vi "Pos_Calculate Random Location.vi"(8 "Error":errorcluster, 9 "Window Size":i16, 10 "Border":i16, 11 "Max Size":i16) -> (0 "Error Out":errorcluster, 2 "Bottom Right Out":i16, 3 "Top Left Out":i16)   [LabVIEW 2015]
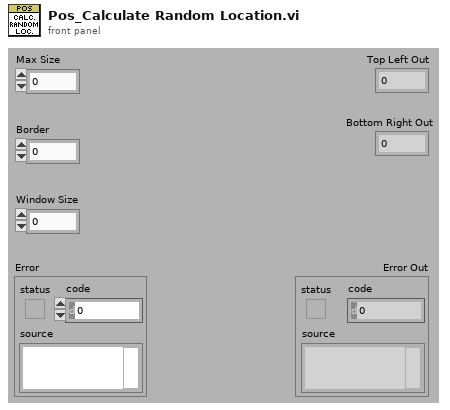
[diagram p1: front panel]
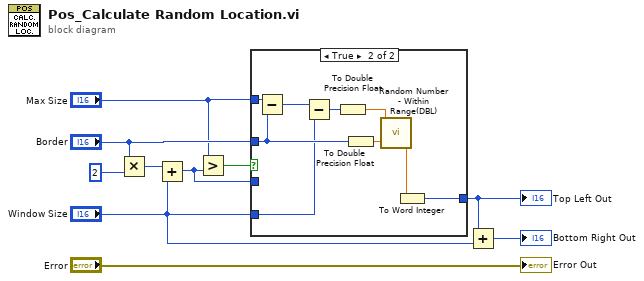
[diagram p0: block diagram]
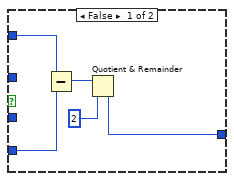
[diagram p2: hidden frame]
diagram:
  n1 = Multiply(x="Border", y=i16 2) -> (x*y=w8:i16)
  n2 = Add(x=w8, y="Window Size") -> (x+y=w4:i16)
  n3 = Greater?(x="Max Size", y=w4) -> (0:w7:bool)
  n4 = case shown="True" w7 {
    tunnel: "Border" -> [_ w22]
    tunnel: "Max Size" -> [w15 w23]
    tunnel: "Window Size" -> [w14 w20]
    tunnel: [w11 w16] -> w2
    tunnel: w4 -> [_ _]
    frame False {
      n5 = Subtract(x=w15, y=w14) -> (x-y=w13:i16)
      n6 = Quotient & Remainder(x=w13, y=i16 2) -> (floor(x/y)=w11:i16)  [unwired: 1 out]
    }
    frame True {
      n7 = Subtract(x=w23, y=w22) -> (x-y=w21:i16)
      n8 = Subtract(x=w21, y=w20) -> (x-y=w19:i16)
      n9 = To Double Precision Float(number=w19) -> (double precision float=w18:dbl)
      n10 = To Double Precision Float(number=w22) -> (double precision float=w24:dbl)
      n11 = call "Random Number - Within Range(DBL).vi"("High (1.00)"=w18, "Low (0.00)"=w24) -> ("Random Number"=w17:dbl)  [unwired: 3 in]
      n12 = To Word Integer(number=w17) -> (16bit integer=w16:i16)
    }
  }
  "Top Left Out" <- w2
  n13 = Add(x=w2, y="Window Size") -> (x+y=→"Bottom Right Out":i16)
  "Error Out" <- "Error"
